vi "LJLogM.vi"() -> ()   [LabVIEW 2026]
uses:
  Common Logger Controls/Device Open Config Cluster.ctl
  Common Logger Controls/Channel Setup.ctl
  Common Logger Controls/Currently Opened Device Params.ctl
  Common Logger Controls/Row Modification Options.ctl
  Common Logger Controls/Program Config Cluster.ctl
panel:
  in  "# Channels":i32=4 min=1 max=96
  in  "Row Modification Options":T1 {"Row #" min=0 max=95}
  in  "Channel Setup":T2={"Name"=["AIN0", "AIN1", "AIN2", "AIN3", "AIN4", "AIN5", "AIN6", "AIN7", "AIN8", "AIN9", "AIN10", "AIN11", "AIN12", "AIN13", "AIN14", "AIN15"], "", "Scaling Equation"=["y=a", "y=b", "y=c", "y=d", "y=e", "y=f", "y=g", "y=h", "y=i", "y=j", "y=k", "y=l", "y=m", "y=n", "y=o", "y=p"], "", "Graph?"=[TRUE, TRUE, TRUE, TRUE, FALSE, FALSE, FALSE, FALSE, FALSE, FALSE, FALSE, FALSE, FALSE, FALSE, FALSE, FALSE]}
  out "Currently Opened Device Params":T3={"Device Type"="ANY", "Connection Type"="ANY", "Serial Number"=0}
  out "Open Configs":T4
  in  "Log Every N Scans":i32=1 min=1 max=2000000000
  in  "Data File Prefix":string="data"
  in  "Log To File":bool
  out "Open Config Name":string
  in  "Select New Configs":bool
  out "App Name":string
  out "Program Config Name":string="LJLogM.cfg"
  out "Actual ms Per Scan":i32
  out "Scan Number":i32
  in  "Scan Interval (ms)":u32=500
  in  "Max File Size (Bytes)":i32=1048576 min=1 max=2000000000
  out "Waveform Graph":cluster{dbl, dbl, dbl[][]}(graph)={0.0, 0.5, []}
  in  "# Scans On Graph":i32=1000 min=0
  in  "exit":bool
  out "Current Data File":path=path "None"
  out "Error Message":string="No Error"
  # "Name"
  # "Raw Value"
  # "Scaling Equation"
  # "Scaled Value"
  # "Graph?"
  # "The raw value for each row corresponds to a scaling variable:"
  # "row 0-15   -->  \"a\"-\"p\""
  # "row 16-31 -->  \"a2\"-\"p2\""
  # "row 32-47 -->  \"a3\"-\"p3\""
  # "row 48-63 -->  \"a4\"-\"p4\""
  # "row 64-79 -->  \"a5\"-\"p5\""
  # "row 80-96 -->  \"a6\"-\"p6\""
  # "The scaled value for a row is represented by the variable  \"y\" in the row's scaling equation."
  # "If your scaling  equation has an error, the scaled value will be zero."
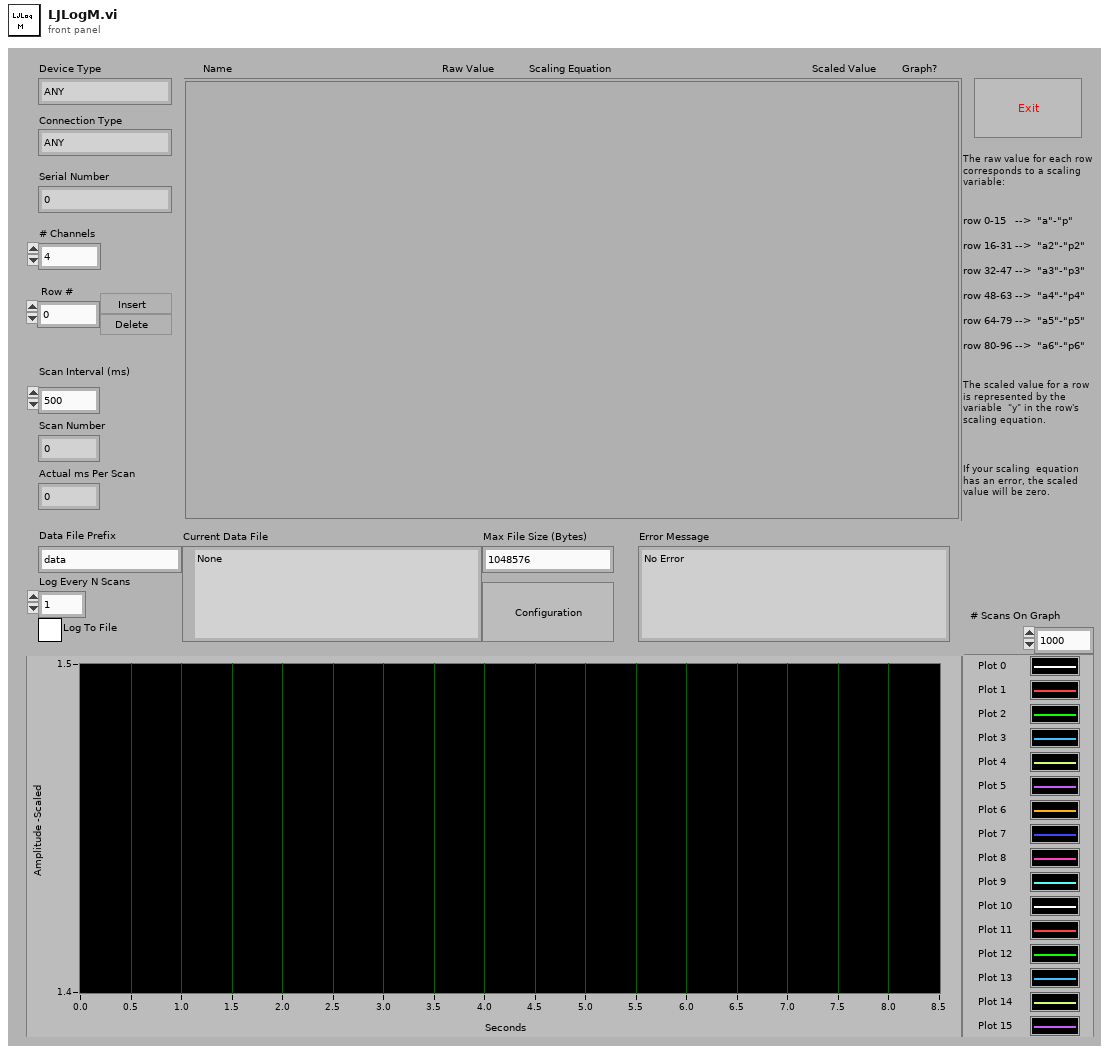
[diagram p1: front panel]
types:
  T1 = typedef "Row Modification Options.ctl" = cluster{" Row #":i32, "Delete Row":bool, "Insert Row":bool}
  T2 = typedef "Channel Setup.ctl" = cluster{"Name":string[], string, "Scaling Equation":string[], string, "Graph?":bool[]}
  T3 = typedef "Currently Opened Device Params.ctl" = cluster{"Device Type":string, "Connection Type":string, "Serial Number":i32}
  T4 = typedef "Device Open Config Cluster.ctl" = cluster{"Open Config Device Type":string, "Open Config Connection Type":string, "Open Config Identifier":string}
  T5 = typedef "Program Config Cluster.ctl" = cluster{"Data File Prefix":string, "Scan Rate (Hz)":dbl, "Graph History":i32, "# Channels":i32, "Disable Scaling":bool, "Max File Size (Bytes)":i32, "Channel Setup":T2, "Interval (ms)":u32, "Write To File":bool, "Log Every n Scans":i32}
  T6 = enum16{"Initialization", "Data Acquisition", "Shutdown", "Reconfiguration"}
  T7 = enum16{"Initialization", "Data Acquisition", "Shutdown"}
  T8 = cluster{"Name":string[], string, "Scaling Equation":string[], string, "Graph?":bool[]}
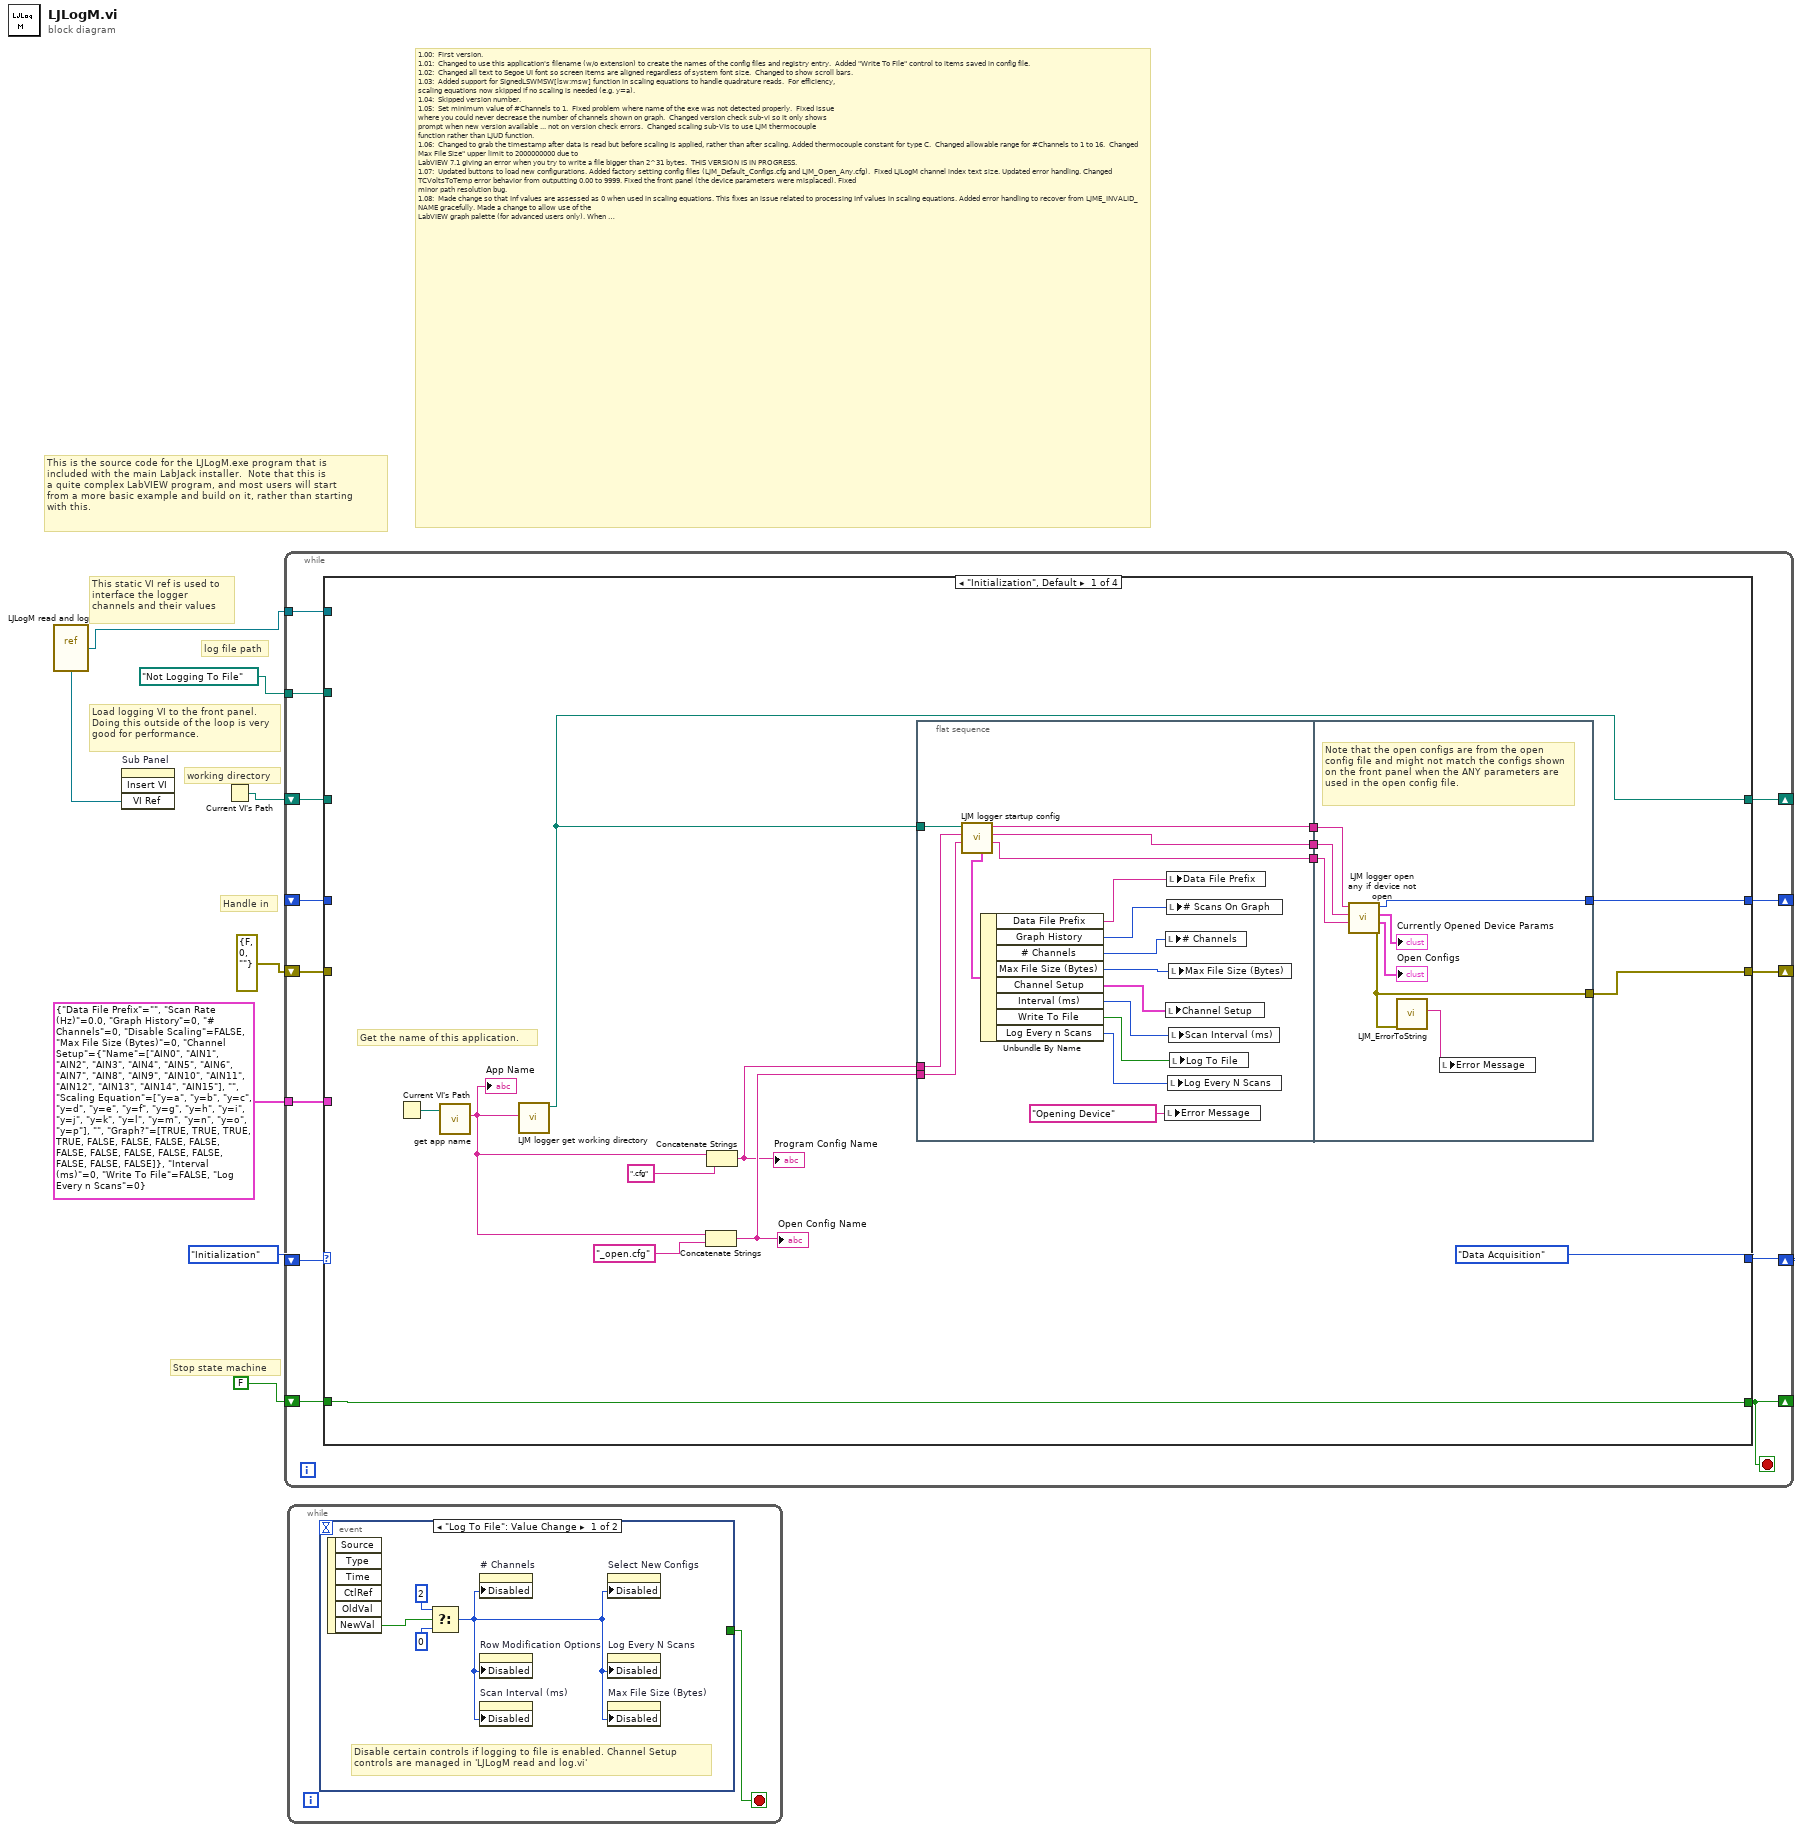
[diagram p0: block diagram]
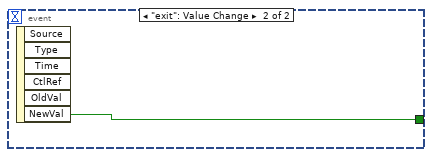
[diagram p2: hidden frame]
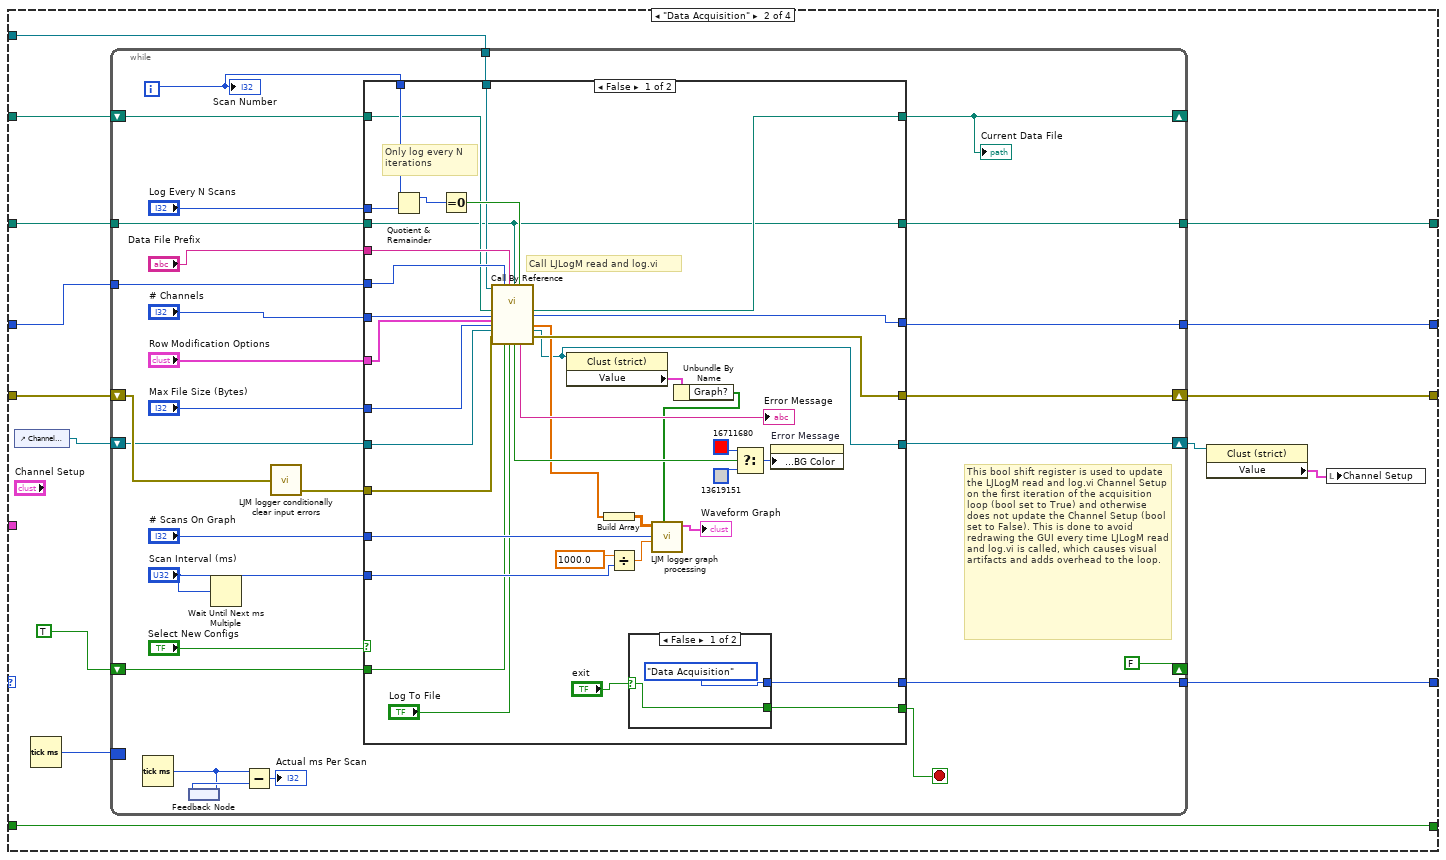
[diagram p3: hidden frame]
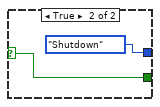
[diagram p4: hidden frame]
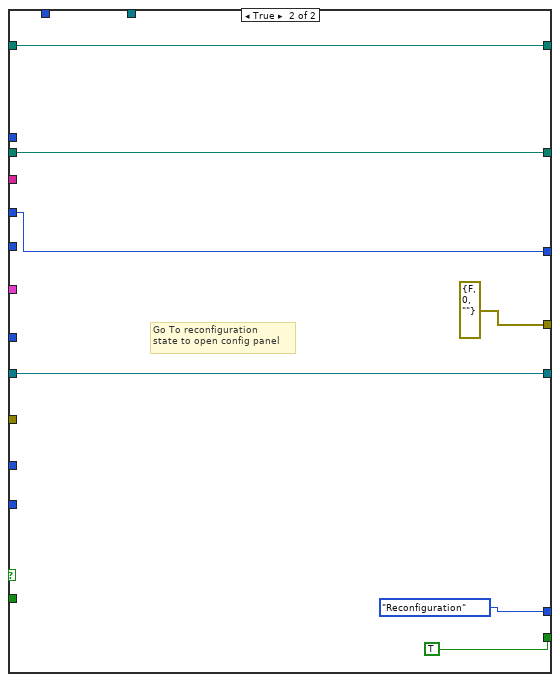
[diagram p5: hidden frame]
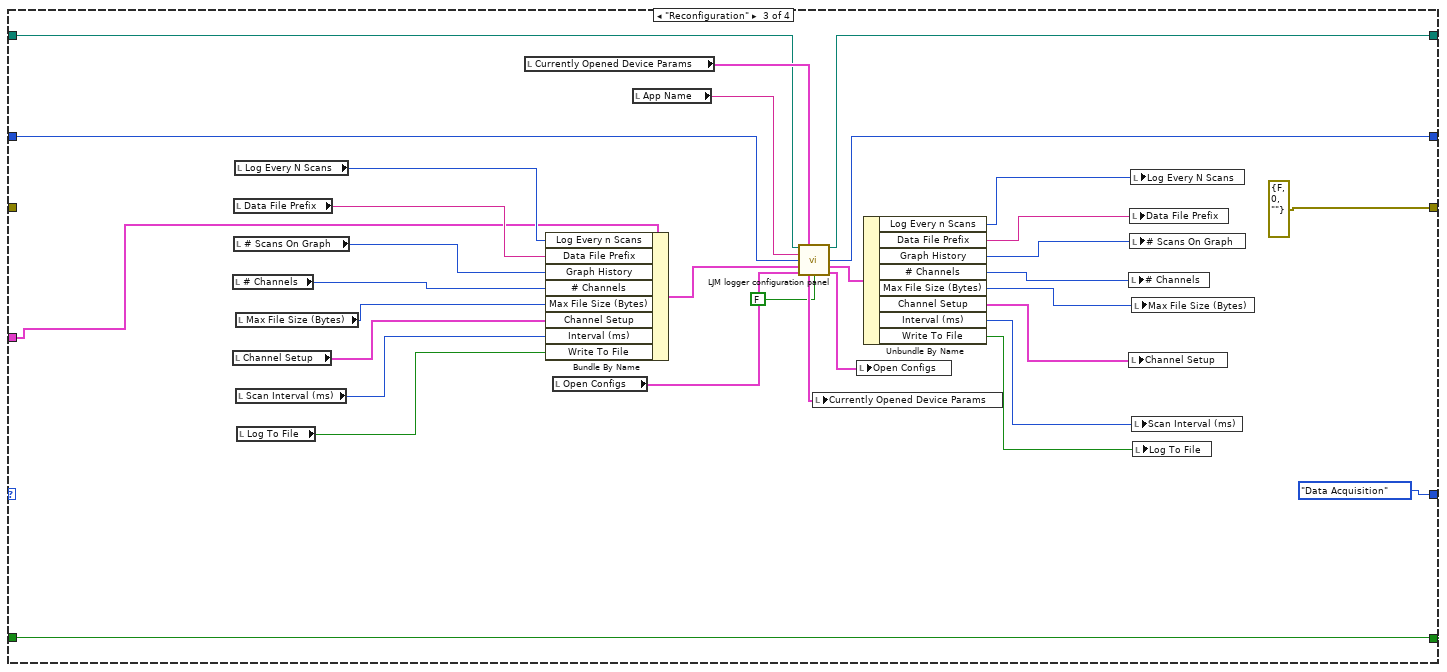
[diagram p6: hidden frame]
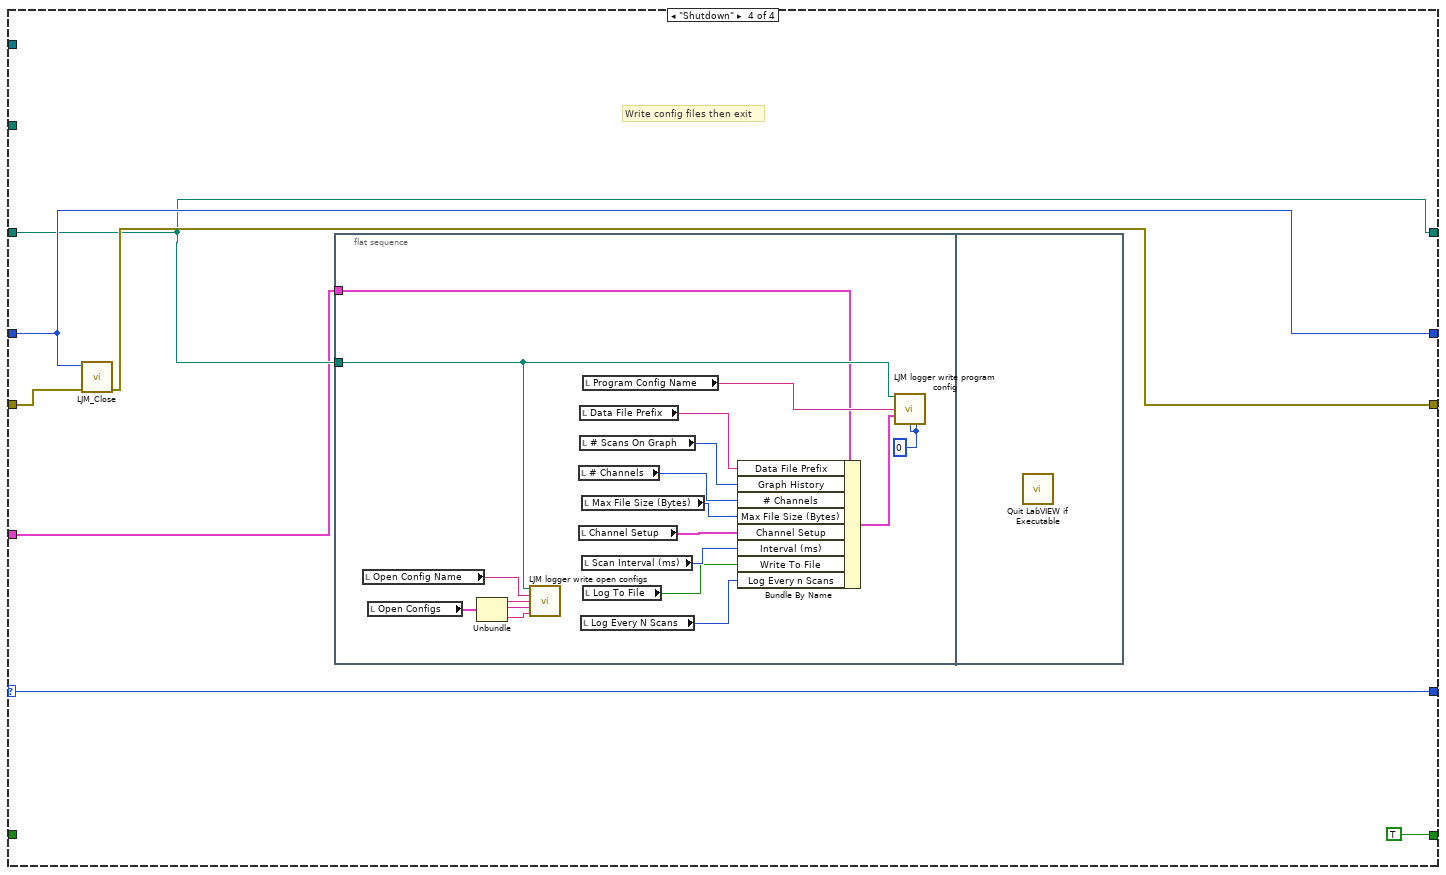
[diagram p7: hidden frame]
diagram:
  # "This static VI ref is used to interface the logger channels and their values"
  # "Load logging VI to the front panel. Doing this outside of the loop is very good for performance."
  # "Stop state machine"
  # "working directory"
  # "log file path"
  # "Handle in"
  # "This is the source code for the LJLogM.exe program that is\nincluded with the main LabJack installer.  Note that this is \na quite complex LabVIEW program, and most users will start\nfrom a more basic example and build on it, rather than starting\nwith this."
  # "1.00:  First version.\n1.01:  Changed to use this application's filename (w/o extension) to create the names of the config files and registry entry.  Added \"Write To File\" control to items saved in config file.\n1.02:  Changed all text to Segoe UI font so screen items are aligned regardless of system font size.  Changed to show scroll bars.\n1.03:  Added support for SignedLSWMSW[lsw:msw] function in scaling equations to handle quadrature reads.  For efficiency,\nscaling equations now skipped if no scaling is needed (e.g. y=a).\n1.04:  Skipped version number.\n1.05:  Set minimum value of #Channels to 1.  Fixed problem where name of the exe was not detected properly.  Fixed issue\nwhere you could never decrease the number of channels shown on graph.  Changed version check sub-vi so it only shows\nprompt when new version available ... not on version check errors.  Changed scaling sub-VIs to use LJM thermocouple\nfunction rather than LJUD function.\n1.06:  Changed to grab the timestamp after data is read but before scaling is applied, rather than after scaling. Added thermocouple constant for type C.  Changed allowable range for #Channels to 1 to 16.  Changed Max File Size\" upper limit to 2000000000 due to\nLabVIEW 7.1 giving an error when you try to write a file bigger than 2^31 bytes.  THIS VERSION IS IN PROGRESS.\n1.07:  Updated buttons to load new configurations. Added factory setting config files (LJM_Default_Configs.cfg and LJM_Open_Any.cfg).  Fixed LJLogM channel index text size. Updated error handling. Changed TCVoltsToTemp error behavior from outputting 0.00 to 9999. Fixed the front panel (the device parameters were misplaced). Fixed\nminor path resolution bug.\n1.08:  Made change so that Inf values are assessed as 0 when used in scaling equations. This fixes an issue related to processing Inf values in scaling equations. Added error handling to recover from LJME_INVALID_NAME gracefully. Made a change to allow use of the\nLabVIEW graph palette (for advanced users only). When set to visible, the palette will be in the bottom right corner of the LJLogM graph. \n1.09:  Fixed SignedMSWLSW scaling equation functionality. This was previously returning an unsigned 32-bit integer representation. It now returns a signed 32-bit integer representation.\n1.10:  Reworked configs including adding a config panel. Moved 'Change Working Directory'. Refactored write to file functionality. Refactored diagram. Added scaling equation error messaging. Renamed 'experiment' config 'program' config. Added register write functionality to configuration panel. Increased front panel text size, changed font to Arial (monospace), and set the minimum panel size. Added 'Log Every n Scans' control. Added support for 96 channels.  Added logger row modification controls. Note: program configs with 96 channels in v1.10 would not be recognized as valid in v1.09\n1.11:  Made minor Visual tweaks to the front panel. Made optimizations to scaling equation processing and front panel responsiveness.\n1.12: If a config file does not exist, load defaults without warning the user. Usually if the config file does not exist it means this is the first time running the program, and we do not want new users to see a warning about the config not existing. Rearranged logger graph palettes on the front panel."
  n1 = vi-ref "LJLogM read and log.vi"() -> ("vi reference"=w2:refnum<vi>)
  n2 = invoke on="Sub Panel" class="SubPnl" method="Insert VI"("VI Ref"=w2) -> ()  [unwired: 3 in, 4 out]
  n3 = Current VI's Path() -> (path=w4:path)
  n4 = while {
    shift-right: [w20] -> _
    shift-left: T6."Initialization" -> [w19]
    shift-right: [w18] -> _
    shift-left: w4 -> [w9]
    shift-right: [w16] -> _
    shift-left: errorcluster {"status"=FALSE, "code"=0, "source"=""} ("error out") -> [w15]
    shift-right: [w17] -> _
    shift-left: _ -> [w14]
    tunnel: path "Not Logging To File" ("y") -> [w13]
    shift-right: [w11] -> _
    shift-left: FALSE -> [w12]
    tunnel: w2 -> [w10]
    tunnel: T5 {"Data File Prefix"="", "Scan Rate (Hz)"=0.0, "Graph History"=0, "# Channels"=0, "Disable Scaling"=FALSE, "Max File Size (Bytes)"=0, "Channel Setup"={"Name"=["AIN0", "AIN1", "AIN2", "AIN3", "AIN4", "AIN5", "AIN6", "AIN7", "AIN8", "AIN9", "AIN10", "AIN11", "AIN12", "AIN13", "AIN14", "AIN15"], "", "Scaling Equation"=["y=a", "y=b", "y=c", "y=d", "y=e", "y=f", "y=g", "y=h", "y=i", "y=j", "y=k", "y=l", "y=m", "y=n", "y=o", "y=p"], "", "Graph?"=[TRUE, TRUE, TRUE, TRUE, FALSE, FALSE, FALSE, FALSE, FALSE, FALSE, FALSE, FALSE, FALSE, FALSE, FALSE, FALSE]}, "Interval (ms)"=0, "Write To File"=FALSE, "Log Every n Scans"=0} ("Program Configs") -> [w8]
    stop <- w11 stop-if-true
    n5 = case shown="\"Initialization\", Default" w19 {
      selector: w19 -> [_ _ _ w184]
      tunnel: [T7."Data Acquisition" w64 T6."Data Acquisition" w184] -> w20
      tunnel: [w23 w66 w156 TRUE] -> w11
      tunnel: [w22 w67 w150 w183] -> w18
      tunnel: [w26 w68 w177 w187] -> w17
      tunnel: [w25 w69 errorcluster {"status"=FALSE, "code"=0, "source"=""} ("error out") w186] -> w16
      tunnel: w15 -> [_ w70 _ w188]
      tunnel: w14 -> [_ w71 w179 w187]
      tunnel: w13 -> [_ w73 _ _]
      tunnel: w12 -> [w23 w66 w156 _]
      tunnel: w10 -> [_ w62 _ _]
      tunnel: w9 -> [_ w65 w151 w183]
      tunnel: w8 -> [_ _ w153 w182]
      frame "Initialization", Default {
        # "Get the name of this application."
        n6 = Current VI's Path() -> (path=w24:path)
        n7 = call "get app name.vi"("Current VI's Path"=w24) -> ("App Name Without Extension"=w29:string)  [unwired: 4 in, 2 out]
        "App Name" <- w29
        n8 = call "LJM logger get working directory.vi"("Application Name"=w29) -> ("Working Directory"=w22:path)  [unwired: 9 in, 1 out]
        n9 = Concatenate Strings(w29, "_open.cfg" ("string")) -> (w30:string)
        "Open Config Name" <- w30
        n10 = Concatenate Strings(w29, ".cfg" ("string")) -> (w21:string)
        "Program Config Name" <- w21
        n11 = flat-sequence {
          tunnel: w22 -> [w48]
          tunnel: w21 -> [w50]
          tunnel: w30 -> [w49]
          tunnel: [w47] -> w33
          tunnel: [w46] -> w32
          tunnel: [w45] -> w31
          tunnel: [w56] -> w25
          tunnel: [w57] -> w26
          tunnel: w33 -> [w55]
          tunnel: w32 -> [w54]
          tunnel: w31 -> [w53]
          frame #0 {
            n12 = call "LJM logger startup config.vi"("Device Open Config Name"=w49, "Program Config Name"=w50, "Working Directory"=w48) -> ("Open Config Identifier"=w45:string, "Open Config ConnectionType"=w46:string, "Open Config Device Type"=w47:string, "Program Configs"=w38:T5)  [unwired: 3 in]
            n13 = Unbundle By Name(w38) -> ("Data File Prefix"=w37:string, "Graph History"=w44:i32, "# Channels"=w43:i32, "Max File Size (Bytes)"=w42:i32, "Channel Setup"=w35:T2, "Interval (ms)"=w41:u32, "Write To File"=w40:bool, "Log Every n Scans"=w39:i32)
            n14 = local write "Error Message"("Opening Device" ("source")) -> ()
            n15 = local write "# Channels"(w43) -> ()
            n16 = local write "Channel Setup"(w35) -> ()
            n17 = local write "Data File Prefix"(w37) -> ()
            n18 = local write "# Scans On Graph"(w44) -> ()
            n19 = local write "Log Every N Scans"(w39) -> ()
            n20 = local write "Max File Size (Bytes)"(w42) -> ()
            n21 = local write "Scan Interval (ms)"(w41) -> ()
            n22 = local write "Log To File"(w40) -> ()
          }
          frame #1 {
            # "Note that the open configs are from the open config file and might not match the configs shown on the front panel when the ANY parameters are used in the open config file."
            n23 = call "LJM logger open any if device not open.vi"("Open Config Identifier"=w53, "Open Config Connection Type"=w54, "Open Config DeviceType"=w55) -> ("error out"=w56:errorcluster, "Open Configs"=→"Open Configs":T4, "Currently Opened Device Params"=→"Currently Opened Device Params":T3, "Handle Out"=w57:i32)  [unwired: 5 in]
            n24 = call "LJM_ErrorToString.vi"("error in"=w56) -> ("String"=w58:string)  [unwired: 10 in]
            n25 = local write "Error Message"(w58) -> ()
          }
        }
      }
      frame "Data Acquisition" {
        n26 = control-ref of="Channel Setup"() -> (w63:refnum<vi>)
        n27 = Tick Count (ms)() -> (millisecond timer value=w72:u32)
        n28 = while {
          shift-right: [w89] -> w69
          shift-left: w70 -> [w99]
          shift-right: [w74] -> _
          shift-left: w73 -> [w77]
          tunnel: w62 -> [w90]
          tunnel: [w87] -> w64
          tunnel: w71 -> [w96]
          tunnel: [w84] -> w68
          tunnel: w65 -> [w97]
          tunnel: [w82] -> w67
          shift-right: [FALSE ("Reconfig Channel Config")] -> _
          shift-left: TRUE ("Reconfig Channel Config") -> [w81]
          shift-right: [w79] -> w60
          shift-left: w63 -> [w86]
          border: w72 -> [_]
          i -> [w76]
          stop <- w88 stop-if-true
          # "This bool shift register is used to update the LJLogM read and log.vi Channel Setup on the first iteration of the acquisition loop (bool set to True) and otherwise does not update the Channel Setup (bool set to False). This is done to avoid redrawing the GUI every time LJLogM read and log.vi is called, which causes visual artifacts and adds overhead to the loop."
          n29 = Tick Count (ms)() -> (millisecond timer value=w100:u32)
          n30 = feedback-in #1(w100) -> ()
          n31 = feedback #1() -> (w101:u32)
          n32 = Wait Until Next ms Multiple(millisecond multiple="Scan Interval (ms)") -> ()  [unwired: 1 out]
          n33 = Subtract(x=w100, y=w101) -> (x-y=→"Actual ms Per Scan":u32)
          n34 = call "LJM logger conditionally clear input errors.vi"("error in"=w99) -> ("error out"=w95:errorcluster)
          n35 = case shown="False" "Select New Configs" {
            tunnel: w97 -> [w106 w144]
            tunnel: w96 -> [w122 w147]
            tunnel: [w117 w147] -> w84
            tunnel: [w118 errorcluster {"status"=FALSE, "code"=0, "source"=""} ("error out")] -> w89
            tunnel: w95 -> [w119 _]
            tunnel: "# Channels" -> [w120 _]
            tunnel: "Scan Interval (ms)" -> [w108 _]
            tunnel: "Max File Size (Bytes)" -> [w110 _]
            tunnel: "# Scans On Graph" -> [w113 _]
            tunnel: "Data File Prefix" -> [w123 _]
            tunnel: "Log Every N Scans" -> [w124 _]
            tunnel: [w126 T6."Reconfiguration"] -> w87
            tunnel: w77 -> [w116 w146]
            tunnel: [w115 w146] -> w74
            tunnel: w76 -> [w125 _]
            tunnel: w90 -> [w121 _]
            tunnel: [w114 TRUE] -> w88
            tunnel: w81 -> [w103 _]
            tunnel: w86 -> [w111 w143]
            tunnel: [w106 w144] -> w82
            tunnel: "Row Modification Options" -> [w104 _]
            tunnel: [w102 w143] -> w79
            frame False {
              # "Call LJLogM read and log.vi"
              # "Only log every N iterations"
              n36 = Quotient & Remainder(x=w125, y=w124) -> (x-y*floor(x/y)=w127:i32)  [unwired: 1 out]
              n37 = Equal To 0?(x=w127) -> (x = 0?=w136:bool)
              n38 = call-by-ref "?"(reference=w121, "Data File Reference In"=w116, "# Channels"=w120, "Row Modification Options"=w104, "Max File Size (Bytes)"=w110, "Channel Setup Reference In"=w111, "Error In"=w119, "Handle In"=w122, "Update Channel Ref"=w103, "Data File Prefix"=w123, "Write to file Selected?"="Log To File", "Working Directory"=w106, "Is Log Interval?"=w136) -> ("Error Message Status"=w134:bool, "Error Message"=→"Error Message":string, "Data File Reference Out"=w115:path, "Handle Out"=w117:i32, "Scaled Data"=w109:dbl[], "Channel Setup Reference Out"=w102:refnum<vi>, "(LJM) Error Out"=w118:errorcluster)  [unwired: 1 in, 3 out]
              n39 = property class="Clust (strict)"(reference=w102) -> ("Value"=w107:T8)  [unwired: 1 in, 2 out]
              n40 = Build Array(w109) -> (w137:dbl[][])
              n41 = Divide(x=1000.0, y=w108) -> (x/y=w132:dbl)
              n42 = case shown="False" "exit" {
                selector: "exit" -> [w140 w141]
                tunnel: [T6."Data Acquisition" T6."Shutdown"] -> w126
                tunnel: [w140 w141] -> w114
                frame False {
                }
                frame True {
                }
              }
              n43 = Unbundle By Name(w107) -> ("Graph?"=w112:bool[])
              n44 = call "LJM logger graph processing.vi"("Graph?"=w112, "Scan Rate"=w132, "Graph History (# scans)"=w113, "Scaled Data"=w137) -> ("Graph Data"=→"Waveform Graph":cluster{dbl, dbl, dbl[][]})  [unwired: 7 in]
              n45 = Select(t=u32 16711680, s=w134, f=u32 13619151) -> (s? t:f=w128:u32)
              n46 = property on="Error Message" class="Str"("Text.Text Colors:BG Color"=w128) -> ()  [unwired: 2 in, 2 out]
            }
            frame True {
              # "Go To reconfiguration\nstate to open config panel"
            }
          }
          "Current Data File" <- w74
          "Scan Number" <- w76
        }
        n47 = property class="Clust (strict)"(reference=w60) -> ("Value"=w59:T8)  [unwired: 1 in, 2 out]
        n48 = local write "Channel Setup"(w59) -> ()
      }
      frame "Reconfiguration" {
        n49 = local read "# Channels"() -> (w175:i32)
        n50 = local read "Channel Setup"() -> (w174:T2)
        n51 = local read "Data File Prefix"() -> (w180:string)
        n52 = local read "# Scans On Graph"() -> (w176:i32)
        n53 = local read "Log Every N Scans"() -> (w181:i32)
        n54 = local read "Max File Size (Bytes)"() -> (w173:i32)
        n55 = local read "Scan Interval (ms)"() -> (w172:u32)
        n56 = local read "Log To File"() -> (w171:bool)
        n57 = local read "Currently Opened Device Params"() -> (w167:T3)
        n58 = Bundle By Name(cluster=w153, "Log Every n Scans"=w181, "Data File Prefix"=w180, "Graph History"=w176, "# Channels"=w175, "Max File Size (Bytes)"=w173, "Channel Setup"=w174, "Interval (ms)"=w172, "Write To File"=w171) -> (w165:T5)
        n59 = local read "Open Configs"() -> (w168:T4)
        n60 = local read "App Name"() -> (w170:string)
        n61 = call "LJM logger configuration panel.vi"("Working Directory"=w151, "Current Device Connection In"=w167, "App name"=w170, "Handle In"=w179, "Program Configs"=w165, "Device Open Params In"=w168, "Streaming App?"=FALSE) -> ("Working Directory Out"=w150:path, "Handle Out"=w177:i32, "Program Configs Out"=w164:T5, "Current Device Connection Out"=w166:T3, "Device Open Params Out"=w169:T4)  [unwired: 4 in]
        n62 = local write "Currently Opened Device Params"(w166) -> ()
        n63 = local write "Open Configs"(w169) -> ()
        n64 = Unbundle By Name(w164) -> ("Log Every n Scans"=w158:i32, "Data File Prefix"=w159:string, "Graph History"=w162:i32, "# Channels"=w154:i32, "Max File Size (Bytes)"=w163:i32, "Channel Setup"=w155:T2, "Interval (ms)"=w161:u32, "Write To File"=w160:bool)
        n65 = local write "# Channels"(w154) -> ()
        n66 = local write "Channel Setup"(w155) -> ()
        n67 = local write "Data File Prefix"(w159) -> ()
        n68 = local write "# Scans On Graph"(w162) -> ()
        n69 = local write "Log Every N Scans"(w158) -> ()
        n70 = local write "Max File Size (Bytes)"(w163) -> ()
        n71 = local write "Scan Interval (ms)"(w161) -> ()
        n72 = local write "Log To File"(w160) -> ()
      }
      frame "Shutdown" {
        # "Write config files then exit"
        n73 = call "LJM_Close.vi"("error in"=w188, "Handle"=w187) -> ("error out"=w186:errorcluster)  [unwired: 9 in]
        n74 = flat-sequence {
          tunnel: w183 -> [w191]
          tunnel: w182 -> [w189]
          frame #0 {
            w190 = u8 0 ("Resolution")
            n75 = local read "Open Config Name"() -> (w202:string)
            n76 = local read "Open Configs"() -> (w206:T4)
            n77 = Unbundle(w206) -> ("Open Config Device Type"=w203:string, "Open Config Connection Type"=w204:string, "Open Config Identifier"=w205:string)
            n78 = call "LJM logger write open configs.vi"("Working Directory"=w191, "Open Config Filename"=w202, "DeviceType"=w203, "ConnectionType"=w204, "Identifier"=w205) -> ()  [unwired: 10 in, 1 out]
            n79 = local read "# Channels"() -> (w197:i32)
            n80 = local read "Channel Setup"() -> (w192:T2)
            n81 = local read "Data File Prefix"() -> (w199:string)
            n82 = local read "# Scans On Graph"() -> (w198:i32)
            n83 = local read "Log Every N Scans"() -> (w193:i32)
            n84 = local read "Max File Size (Bytes)"() -> (w196:i32)
            n85 = local read "Scan Interval (ms)"() -> (w195:u32)
            n86 = local read "Program Config Name"() -> (w201:string)
            n87 = local read "Log To File"() -> (w194:bool)
            n88 = Bundle By Name(cluster=w189, "Data File Prefix"=w199, "Graph History"=w198, "# Channels"=w197, "Max File Size (Bytes)"=w196, "Channel Setup"=w192, "Interval (ms)"=w195, "Write To File"=w194, "Log Every n Scans"=w193) -> (w200:T5)
            n89 = call "LJM logger write program config.vi"("Working Directory"=w191, "filename"=w201, "Program Configs"=w200, "Resolution"=w190, "SettlingFactor"=w190) -> ()  [unwired: 10 in, 1 out]
          }
          frame #1 {
            n90 = call "Quit LabVIEW if Executable.vi"() -> ()  [unwired: 1 in]
          }
        }
      }
    }
  }
  n91 = while {
    stop <- w207 stop-if-true
    n92 = event shown="[0] \"Log To File\": Value Change" {
      selector: _ -> [_ _]
      dyn-events: _ -> [_ _]
      timeout: _ -> [_ _]
      tunnel: [_ w212] -> w207
      event "Log To File": Value Change {
        # "Disable certain controls if logging to file is enabled. Channel Setup controls are managed in 'LJLogM read and log.vi'"
        n93 = event-data() -> ("NewVal"=w209:bool)  [unwired: 1 in, 5 out]
        n94 = Select(t=u8 2 ("Disabled"), s=w209, f=u8 0 ("Disabled")) -> (s? t:f=w208:u8)
        n95 = property on="# Channels" class="DigNum (strict)"("Disabled"=w208) -> ()  [unwired: 2 in, 2 out]
        n96 = property on="Row Modification Options" class="Clust"("Disabled"=w208) -> ()  [unwired: 2 in, 2 out]
        n97 = property on="Scan Interval (ms)" class="DigNum (strict)"("Disabled"=w208) -> ()  [unwired: 2 in, 2 out]
        n98 = property on="Select New Configs" class="Bool"("Disabled"=w208) -> ()  [unwired: 2 in, 2 out]
        n99 = property on="Log Every N Scans" class="DigNum (strict)"("Disabled"=w208) -> ()  [unwired: 2 in, 2 out]
        n100 = property on="Max File Size (Bytes)" class="DigNum (strict)"("Disabled"=w208) -> ()  [unwired: 2 in, 2 out]
      }
      event "exit": Value Change {
        n101 = event-data() -> ("NewVal"=w212:bool)  [unwired: 1 in, 5 out]
      }
    }
  }
